vi "Test Epochs.vi"() -> ()   [LabVIEW 2013]
uses:
  source/epoch.UTC/Epoch.UTC.lvclass
  source/epoch/Epoch.lvclass
  source/epoch.GPS/Epoch.GPS.lvclass
  source/epoch.UNIX/Epoch.UNIX.lvclass
  source/formatter.iso8601/DateTime.ISO8601.lvclass
  source/formatter.iso8601/ISO8601 Date Formats.ctl
  source/Timestamp Compare Units -- enum.ctl
  source/formatter.iso8601/DateTime.ISO8601.lvclass/DateTime.ISO8601.ctl
  source/isLeapYear (integer).vi
  source/isLeapYear (timestamp).vi
  source/formatter/DateTimeFormatter.lvclass
panel:
  in  "Timestamp":timestamp
  out "Valid RFC3339 Dates":bool
  out "Valid ISO Dates":bool
  out "ISO Week":bool
  out "ISO DateTime (with UTC)":bool
  out "ISO DateTime (no UTC)":bool
  out "Ordinal Date Test":bool[](array[boolean])
  out "is Leap Year?":bool
  out "Weekday Test Vectors":bool[](array[boolean])
  out "ISO8601 DateTime (Week)":string
  out "Not a Timestamp?":bool
  out "ISO8601 DateTime (UTC)":string
  out "ISO8601 DateTime":string
  out "Local = Current Timestamp":bool
  out "Unix Time (s)":i64
  out "Unix = Local":bool
  out "GPS = Local Timestamp":bool
  out "GPS Time (s)":i64
  out "UTC = Local":bool
  out "current system time":timestamp
  out "UTC Time (s)":i64
  out "Fractional Second":dbl format="%#.6f"
  out "Local Time (s)":i64
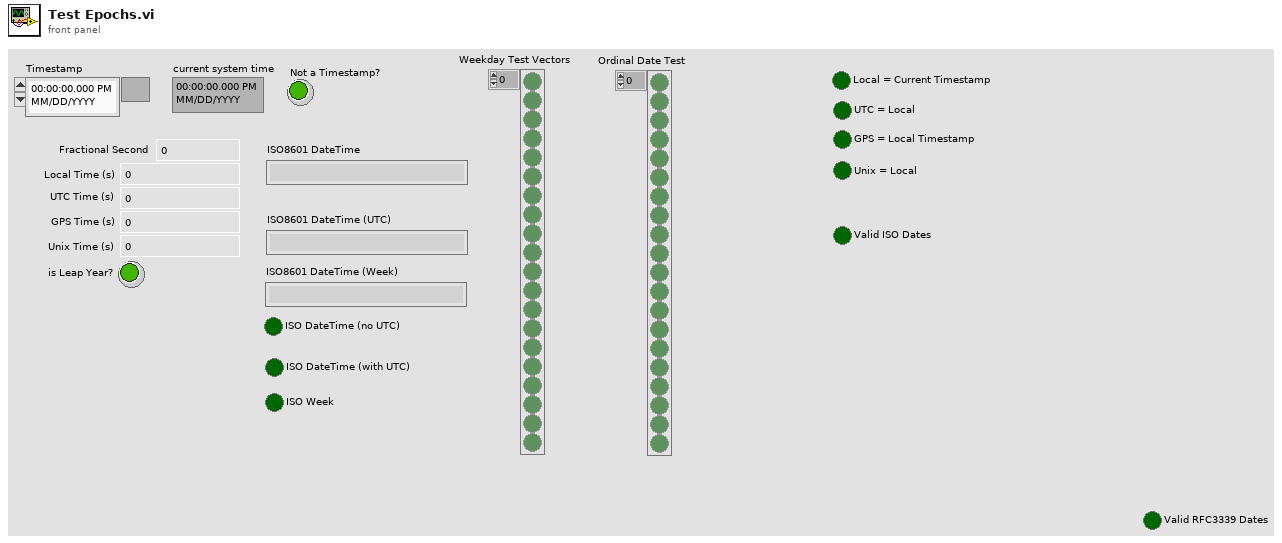
[diagram p1: front panel]
types:
  T1 = typedef "Timestamp Compare Units -- enum.ctl" = enum16{"week", "day", "hour", "minute", "second", "millisecond", "microsecond", "nanosecond"}
  T2 = typedef "ISO8601 Date Formats.ctl" = enum16{"UTC Date-Time", "Date", "Calendar Month", "Week", "Week-Day", "Month-Day", "Ordinal Date"}
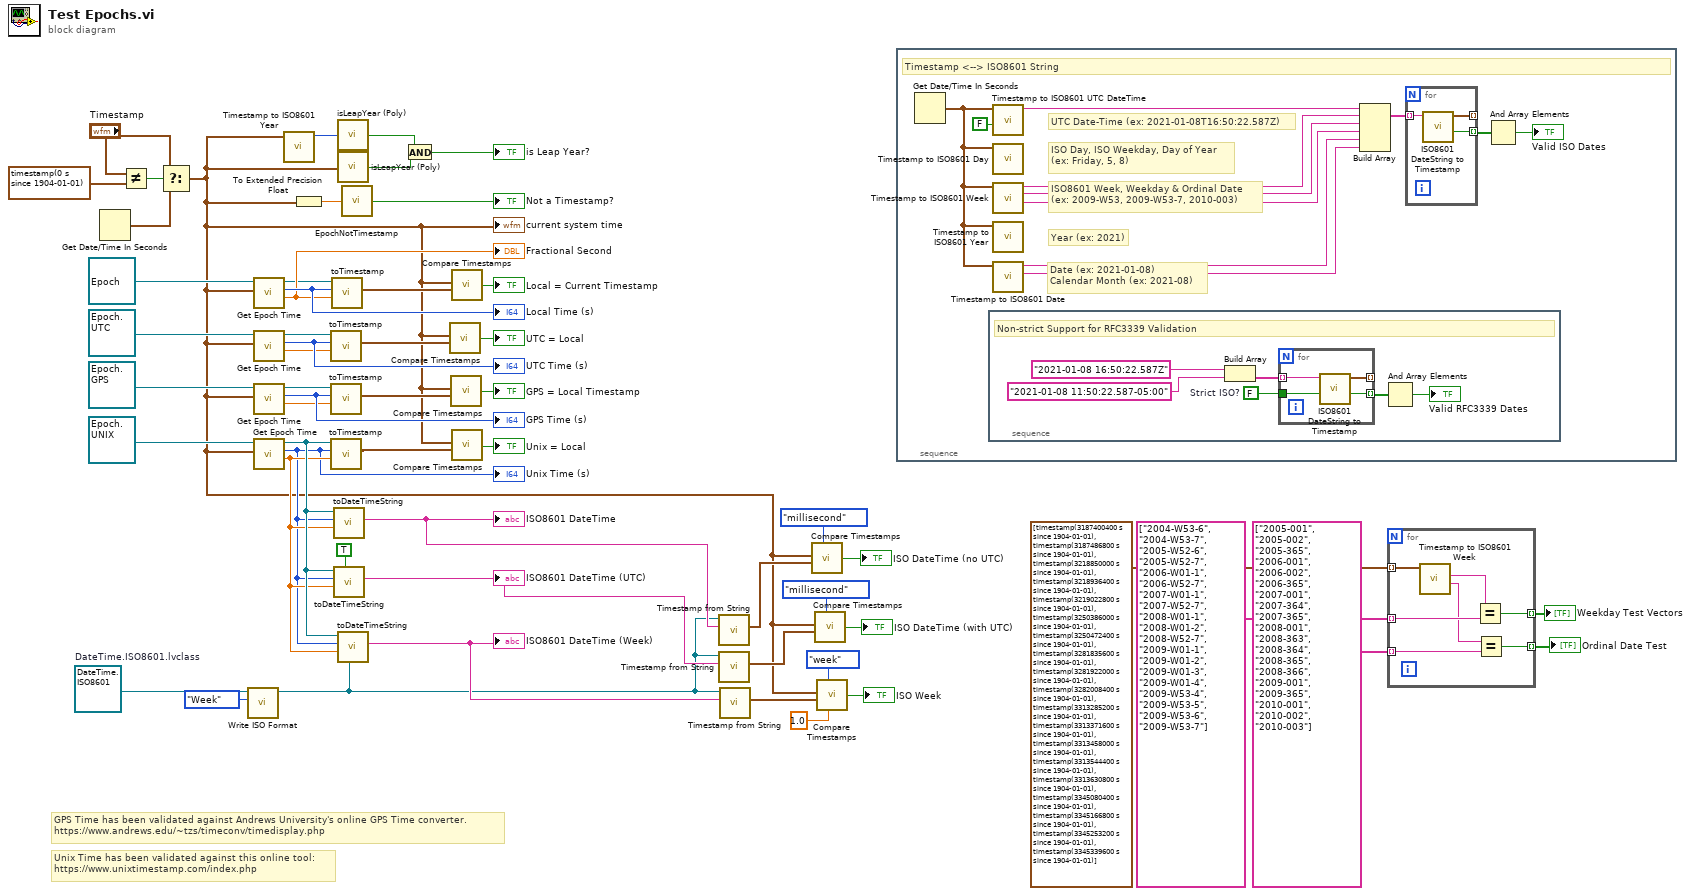
[diagram p0: block diagram]
diagram:
  w36 = refnum<class "DateTime.ISO8601.lvclass"> refnum  # DateTime.ISO8601.lvclass
  # "Unix Time has been validated against this online tool:\nhttps://www.unixtimestamp.com/index.php"
  # "GPS Time has been validated against Andrews University's online GPS Time converter.\nhttps://www.andrews.edu/~tzs/timeconv/timedisplay.php"
  n1 = Get Date/Time In Seconds() -> (seconds since 1Jan1904=w10:timestamp)
  n2 = Not Equal?(x="Timestamp", y=timestamp(0 s since 1904-01-01)) -> (x != y?=w12:bool)
  n3 = Select(t="Timestamp", s=w12, f=w10) -> (s? t:f=w1:timestamp)
  "current system time" <- w1
  n4 = call "Write ISO Format.vi"("ISO Format"=ISO8601_Date_Formats."Week", "DateTime.ISO8601 in"=w36) -> ("DateTime.ISO8601 out"=w13:refnum<class "DateTime.ISO8601.lvclass">)  [unwired: 9 in]
  n5 = call "Get Epoch Time.vi"("Timestamp (now)"=w1, "Epoch (Local)"=refnum<class "Epoch.lvclass"> refnum ("Epoch.lvclass")) -> ("Fractional Second"=w48:dbl, "Epoch Time (s)"=w54:i64, "Epoch out"=w47:refnum<class "Epoch.lvclass">)  [unwired: 7 in]
  "Local Time (s)" <- w54
  "Fractional Second" <- w48
  n6 = call "Get Epoch Time.vi"("Timestamp (now)"=w1, "Epoch (Local)"=refnum<class "Epoch.UTC.lvclass"> refnum ("Epoch.UTC.lvclass")) -> ("Fractional Second"=w49:dbl, "Epoch Time (s)"=w55:i64, "Epoch out"=w50:refnum<class "Epoch.UTC.lvclass">)  [unwired: 7 in]
  "UTC Time (s)" <- w55
  n7 = call "Get Epoch Time.vi"("Timestamp (now)"=w1, "Epoch (Local)"=refnum<class "Epoch.GPS.lvclass"> refnum ("Epoch.GPS.lvclass")) -> ("Fractional Second"=w45:dbl, "Epoch Time (s)"=w52:i64, "Epoch out"=w44:refnum<class "Epoch.GPS.lvclass">)  [unwired: 7 in]
  "GPS Time (s)" <- w52
  n8 = call "Get Epoch Time.vi"("Timestamp (now)"=w1, "Epoch (Local)"=refnum<class "Epoch.UNIX.lvclass"> refnum ("Epoch.UNIX.lvclass")) -> ("Fractional Second"=w39:dbl, "Epoch Time (s)"=w37:i64, "Epoch out"=w40:refnum<class "Epoch.UNIX.lvclass">)  [unwired: 7 in]
  "Unix Time (s)" <- w37
  n9 = call "Timestamp to ISO8601 Year.vi"("Timestamp (now)"=w1) -> ("year"=w30:i32)  [unwired: 9 in, 1 out]
  n10 = To Extended Precision Float(1:w1) -> (0:w42:ext)
  n11 = call-dynamic "toTimestamp.vi"("Fractional Second"=w49, "UTC Time (s)"=w55, "Epoch (UTC)"=w50) -> ("Timestamp"=w6:timestamp)  [unwired: 6 in, 2 out]
  n12 = call-dynamic "toTimestamp.vi"("Fractional Second"=w45, "GPS Time (s)"=w52, "Epoch (GPS)"=w44) -> ("Timestamp"=w2:timestamp)  [unwired: 6 in, 2 out]
  n13 = call-dynamic "toTimestamp.vi"("Fractional Second"=w39, "Unix Time (s)"=w37, "Epoch (Unix)"=w40) -> ("Timestamp"=w3:timestamp)  [unwired: 6 in, 2 out]
  n14 = call-dynamic "toTimestamp.vi"("Fractional Second"=w48, "Epoch Time (s)"=w54, "Epoch (Local)"=w47) -> ("Timestamp"=w7:timestamp)  [unwired: 6 in, 2 out]
  n15 = call "toDateTimeString.vi"("Fractional Second"=w39, "Epoch Time (s)"=w37, "Epoch"=w40) -> ("DateTime string"=w29:string)  [unwired: 6 in, 2 out]
  "ISO8601 DateTime" <- w29
  n16 = call "toDateTimeString.vi"("UTC? (F)"=TRUE, "Fractional Second"=w39, "Epoch Time (s)"=w37, "Epoch"=w40) -> ("DateTime string"=w28:string)  [unwired: 5 in, 2 out]
  "ISO8601 DateTime (UTC)" <- w28
  n17 = call-poly "isLeapYear (Poly).vi"("Year (0: this year)"=w30) -> ("is Leap Year?"=w26:bool)  [unwired: 8 in]
  n18 = call-poly "isLeapYear (Poly).vi"("timestamp (now)"=w1) -> ("is Leap Year?"=w25:bool)  [unwired: 8 in]
  n19 = call "toDateTimeString.vi"("DateTimeFormatter (ISO8601)"=w13, "Fractional Second"=w39, "Epoch Time (s)"=w37, "Epoch"=w40) -> ("DateTime string"=w27:string)  [unwired: 5 in, 2 out]
  "ISO8601 DateTime (Week)" <- w27
  n20 = call "EpochNotTimestamp.vi"("Epoch Time"=w42) -> ("Not a Timestamp?"=→"Not a Timestamp?":bool)  [unwired: 8 in]
  n21 = And(x=w26, y=w25) -> (x .and. y?=→"is Leap Year?":bool)
  n22 = call "Compare Timestamps.vi"("timestamp (1)"=w1, "timestamp (2)"=w6) -> ("Equal?"=→"UTC = Local":bool)  [unwired: 6 in]
  n23 = call "Compare Timestamps.vi"("timestamp (1)"=w1, "timestamp (2)"=w2) -> ("Equal?"=→"GPS = Local Timestamp":bool)  [unwired: 6 in]
  n24 = call "Compare Timestamps.vi"("timestamp (1)"=w1, "timestamp (2)"=w7) -> ("Equal?"=→"Local = Current Timestamp":bool)  [unwired: 6 in]
  n25 = call "Compare Timestamps.vi"("timestamp (1)"=w1, "timestamp (2)"=w3) -> ("Equal?"=→"Unix = Local":bool)  [unwired: 6 in]
  n26 = call "Timestamp from String.vi"("DateTime String"=w29, "DateTimeFormatter in"=w13) -> ("Timestamp"=w21:timestamp)  [unwired: 7 in, 2 out]
  n27 = call "Timestamp from String.vi"("DateTime String"=w28, "DateTimeFormatter in"=w13) -> ("Timestamp"=w20:timestamp)  [unwired: 7 in, 2 out]
  n28 = call "Timestamp from String.vi"("DateTime String"=w27, "DateTimeFormatter in"=w13) -> ("Timestamp"=w18:timestamp)  [unwired: 7 in, 2 out]
  n29 = call "Compare Timestamps.vi"("Unit (ms)"=Timestamp_Compare_Units_--_enum."millisecond" ("Unit (second)"), "timestamp (1)"=w1, "timestamp (2)"=w21) -> ("Equal?"=→"ISO DateTime (no UTC)":bool)  [unwired: 5 in]
  n30 = call "Compare Timestamps.vi"("Unit (ms)"=Timestamp_Compare_Units_--_enum."millisecond" ("Unit (second)"), "timestamp (1)"=w1, "timestamp (2)"=w20) -> ("Equal?"=→"ISO DateTime (with UTC)":bool)  [unwired: 5 in]
  n31 = call "Compare Timestamps.vi"("Unit (ms)"=Timestamp_Compare_Units_--_enum."week" ("Unit (second)"), "timestamp (1)"=w1, "timestamp (2)"=w18, "Resolution (in selected unit)"=1.0) -> ("Equal?"=→"ISO Week":bool)  [unwired: 4 in]
  n32 = stacked-sequence {
    frame #0 {
      # "Date (ex: 2021-01-08)\nCalendar Month (ex: 2021-08)"
      # "Year (ex: 2021)"
      # "ISO8601 Week, Weekday & Ordinal Date\n(ex: 2009-W53, 2009-W53-7, 2010-003)"
      # "ISO Day, ISO Weekday, Day of Year\n(ex: Friday, 5, 8)"
      # "UTC Date-Time (ex: 2021-01-08T16:50:22.587Z)"
      # "Timestamp <--> ISO8601 String"
      n33 = Get Date/Time In Seconds() -> (seconds since 1Jan1904=w67:timestamp)
      n34 = stacked-sequence {
        frame #0 {
          w71 = FALSE  # Strict ISO?
          # "Non-strict Support for RFC3339 Validation"
          n35 = Build Array("2021-01-08 16:50:22.587Z" ("x"), "2021-01-08 11:50:22.587-05:00" ("x")) -> (w74:string[])
          n36 = for {
            tunnel: w74 -> [w78] mode=indexing
            tunnel: [w77] -> w73 mode=indexing
            tunnel: w71 -> [w76]
            tunnel: [w75] -> _ mode=indexing
            n37 = call "ISO8601 DateString to Timestamp.vi"("Strict ISO? (T)"=w76, "ISO8601 Date String"=w78) -> ("valid?"=w77:bool, "Timestamp"=w75:timestamp)  [unwired: 7 in, 1 out]
          }
          n38 = And Array Elements(Boolean array=w73) -> (logical AND=→"Valid RFC3339 Dates":bool)
        }
      }
      n39 = call "Timestamp to ISO8601 UTC DateTime.vi"("UTC? (F)"=FALSE, "Timestamp (now)"=w67) -> ("ISO8601 UTC DateTime"=w66:string)  [unwired: 9 in]
      n40 = call "Timestamp to ISO8601 Day.vi"("Timestamp (now)"=w67) -> ()  [unwired: 8 in, 3 out]
      n41 = call "Timestamp to ISO8601 Week.vi"("Timestamp (now)"=w67) -> ("ISO8601 Ordinal Date"=w63:string, "ISO8601 Weekday"=w64:string, "ISO8601 Week"=w65:string)  [unwired: 8 in]
      n42 = call "Timestamp to ISO8601 Year.vi"("Timestamp (now)"=w67) -> ()  [unwired: 9 in, 2 out]
      n43 = call "Timestamp to ISO8601 Date.vi"("Timestamp (now)"=w67) -> ("ISO8601 Calendar Month"=w61:string, "ISO8601 Date"=w62:string)  [unwired: 9 in]
      n44 = Build Array(w66, w65, w64, w63, w62, w61) -> (w60:string[])
      n45 = for {
        tunnel: w60 -> [w81] mode=indexing
        tunnel: [w80] -> w59 mode=indexing
        tunnel: [w79] -> _ mode=indexing
        n46 = call "ISO8601 DateString to Timestamp.vi"("ISO8601 Date String"=w81) -> ("valid?"=w80:bool, "Timestamp"=w79:timestamp)  [unwired: 8 in, 1 out]
      }
      n47 = And Array Elements(Boolean array=w59) -> (logical AND=→"Valid ISO Dates":bool)
    }
  }
  n48 = for {
    tunnel: timestamp[] [timestamp(3187400400 s since 1904-01-01), timestamp(3187486800 s since 1904-01-01), timestamp(3218850000 s since 1904-01-01), timestamp(3218936400 s since 1904-01-01), timestamp(3219022800 s since 1904-01-01), timestamp(3250386000 s since 1904-01-01), timestamp(3250472400 s since 1904-01-01), timestamp(3281835600 s since 1904-01-01), timestamp(3281922000 s since 1904-01-01), timestamp(3282008400 s since 1904-01-01), timestamp(3313285200 s since 1904-01-01), timestamp(3313371600 s since 1904-01-01), timestamp(3313458000 s since 1904-01-01), timestamp(3313544400 s since 1904-01-01), timestamp(3313630800 s since 1904-01-01), timestamp(3345080400 s since 1904-01-01), timestamp(3345166800 s since 1904-01-01), timestamp(3345253200 s since 1904-01-01), timestamp(3345339600 s since 1904-01-01)] -> [w83] mode=indexing
    tunnel: string[] ["2004-W53-6", "2004-W53-7", "2005-W52-6", "2005-W52-7", "2006-W01-1", "2006-W52-7", "2007-W01-1", "2007-W52-7", "2008-W01-1", "2008-W01-2", "2008-W52-7", "2009-W01-1", "2009-W01-2", "2009-W01-3", "2009-W01-4", "2009-W53-4", "2009-W53-5", "2009-W53-6", "2009-W53-7"] -> [w86] mode=indexing
    tunnel: [w88] -> w33 mode=indexing
    tunnel: string[] ["2005-001", "2005-002", "2005-365", "2006-001", "2006-002", "2006-365", "2007-001", "2007-364", "2007-365", "2008-001", "2008-363", "2008-364", "2008-365", "2008-366", "2009-001", "2009-365", "2010-001", "2010-002", "2010-003"] -> [w85] mode=indexing
    tunnel: [w84] -> w31 mode=indexing
    n49 = call "Timestamp to ISO8601 Week.vi"("Timestamp (now)"=w83) -> ("ISO8601 Ordinal Date"=w82:string, "ISO8601 Weekday"=w87:string)  [unwired: 8 in, 1 out]
    n50 = Equal?(x=w87, y=w86) -> (x = y?=w88:bool)
    n51 = Equal?(x=w82, y=w85) -> (x = y?=w84:bool)
  }
  "Weekday Test Vectors" <- w33
  "Ordinal Date Test" <- w31
